vi "Asset Example.vi"() -> ()   [LabVIEW 2019]
uses:
  <vilib>/Skyline/AssetManagement/Start Utilization (All).vi
  <vilib>/Skyline/AssetManagement/Start Utilization (Single).vi
  <vilib>/Skyline/AssetManagement/NI SystemLink Asset Utilization.lvclass
panel:
  out "Time":u32
  in  "stop":bool
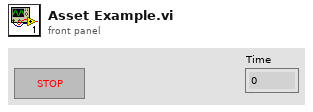
[diagram p1: front panel]
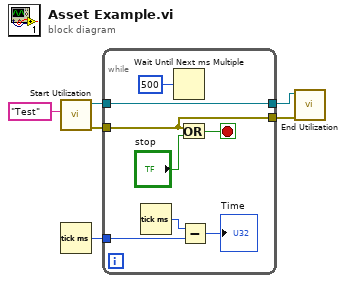
[diagram p0: block diagram]
diagram:
  n1 = call-poly <vilib>:"Start Utilization.vi"("utilization category"="Test") -> ("error out"=w4:errorcluster, "asset utilization"=w5:refnum<class "NI SystemLink Asset Utilization.lvclass">)  [unwired: 9 in]
  n2 = Tick Count (ms)() -> (millisecond timer value=w6:u32)
  n3 = while {
    tunnel: w6 -> [w13]
    tunnel: [w11] -> w2
    tunnel: w5 -> [w11]
    tunnel: w4 -> [w10]
    tunnel: [w10] -> w3
    stop <- w8 stop-if-true
    n4 = Tick Count (ms)() -> (millisecond timer value=w14:u32)
    n5 = Wait Until Next ms Multiple(millisecond multiple=u32 500) -> ()  [unwired: 1 out]
    n6 = Or(x=w10, y="stop") -> (x .or. y?=w8:bool)
    n7 = Subtract(x=w14, y=w13) -> (x-y=→"Time":u32)
  }
  n8 = call <vilib>:"End Utilization.vi"("error in (no error)"=w3, "asset utilization"=w2) -> ()  [unwired: 9 in, 1 out]
